vi "SCM4_MAG_Signaling.vi"() -> ()   [LabVIEW 2018]
panel:
  in  "Setpoint [T]":dbl=0.3 format="%#_4g"
  in  "Slew rate":dbl=0.3 format="%#_4g"
  in  "ico":u16(ring)=1 items=["Field"=1, "Rate"=2]
  # "ico = 1 Field\n       = 2 Rate"
  # "T/min"
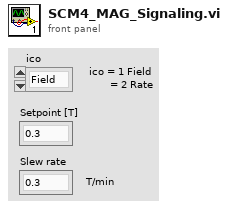
[diagram p1: front panel]
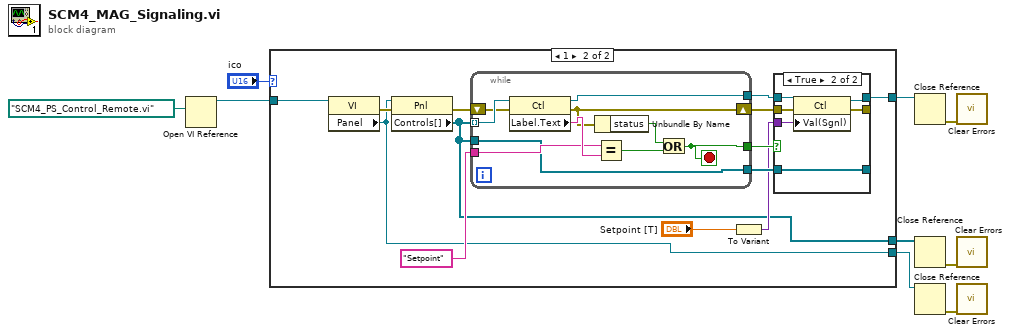
[diagram p0: block diagram]
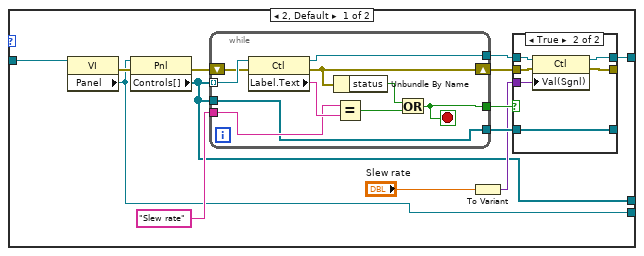
[diagram p2: hidden frame]
diagram:
  n1 = Open VI Reference(vi path=path "SCM4_PS_Control_Remote.vi") -> (vi reference=w7:refnum<vi>)  [unwired: 5 in, 1 out]
  n2 = case shown="1" "ico" {
    tunnel: w7 -> [w13 w45]
    tunnel: [w12 w44] -> w4
    tunnel: [w11 w43] -> w3
    tunnel: [w10 w42] -> w2
    frame 2, Default {
      n3 = property class="VI"(reference=w13) -> (error out=w22:errorcluster, "Panel"=w10:refnum<vi>)  [unwired: 1 in, 1 out]
      n4 = property class="Pnl"(reference=w10, error in=w22) -> (error out=w21:errorcluster, "Controls[]"=w11:refnum<vi>[])  [unwired: 1 out]
      n5 = while {
        tunnel: w11 -> [w41] mode=indexing
        tunnel: "Slew rate" ("Control Name") -> [w39]
        shift-right: [w36] -> w18
        shift-left: w21 -> [w38]
        tunnel: [w37] -> w20
        tunnel: [w33] -> w19
        tunnel: w11 -> [w32]
        tunnel: [w32] -> w17
        stop <- w33 stop-if-true
        n6 = property class="Ctl"(reference=w41, error in=w38) -> (reference out=w37:refnum<vi>, error out=w36:errorcluster, "Label.Text"=w40:string)
        n7 = Unbundle By Name(w36) -> ("status"=w35:bool)
        n8 = Equal?(x=w39, y=w40) -> (x = y?=w34:bool)
        n9 = Or(x=w35, y=w34) -> (x .or. y?=w33:bool)
      }
      n10 = To Variant(anything="Slew rate") -> (Variant=w15:variant)
      n11 = case shown="True" w19 {
        tunnel: w20 -> [w24 w30]
        tunnel: w18 -> [w25 w31]
        tunnel: [w25 w29] -> _
        tunnel: [w24 w28] -> w12
        tunnel: w17 -> [w23 w27]
        tunnel: [w23 w27] -> _
        tunnel: w15 -> [_ w26]
        frame False {
        }
        frame True {
          n12 = property on="Property Node" class="Ctl"(reference=w30, error in=w31, "Val(Sgnl)"=w26) -> (reference out=w28:refnum<vi>, error out=w29:errorcluster)
        }
      }
    }
    frame 1 {
      n13 = property class="VI"(reference=w45) -> (error out=w54:errorcluster, "Panel"=w42:refnum<vi>)  [unwired: 1 in, 1 out]
      n14 = property class="Pnl"(reference=w42, error in=w54) -> (error out=w53:errorcluster, "Controls[]"=w43:refnum<vi>[])  [unwired: 1 out]
      n15 = while {
        tunnel: w43 -> [w73] mode=indexing
        tunnel: "Setpoint" ("Control Name") -> [w71]
        shift-right: [w68] -> w50
        shift-left: w53 -> [w70]
        tunnel: [w69] -> w52
        tunnel: [w65] -> w51
        tunnel: w43 -> [w64]
        tunnel: [w64] -> w49
        stop <- w65 stop-if-true
        n16 = property class="Ctl"(reference=w73, error in=w70) -> (reference out=w69:refnum<vi>, error out=w68:errorcluster, "Label.Text"=w72:string)
        n17 = Unbundle By Name(w68) -> ("status"=w67:bool)
        n18 = Equal?(x=w71, y=w72) -> (x = y?=w66:bool)
        n19 = Or(x=w67, y=w66) -> (x .or. y?=w65:bool)
      }
      n20 = To Variant(anything="Setpoint [T]") -> (Variant=w47:variant)
      n21 = case shown="True" w51 {
        tunnel: w52 -> [w56 w62]
        tunnel: w50 -> [w57 w63]
        tunnel: [w57 w61] -> _
        tunnel: [w56 w60] -> w44
        tunnel: w49 -> [w55 w59]
        tunnel: [w55 w59] -> _
        tunnel: w47 -> [_ w58]
        frame False {
        }
        frame True {
          n22 = property class="Ctl"(reference=w62, error in=w63, "Val(Sgnl)"=w58) -> (reference out=w60:refnum<vi>, error out=w61:errorcluster)
        }
      }
    }
  }
  n23 = Close Reference(reference=w4) -> (error out=w8:errorcluster)  [unwired: 1 in]
  n24 = Close Reference(reference=w3) -> (error out=w6:errorcluster)  [unwired: 1 in]
  n25 = Close Reference(reference=w2) -> (error out=w5:errorcluster)  [unwired: 1 in]
  n26 = call <vilib>:"Clear Errors.vi"("error in (no error)"=w8) -> ()  [unwired: 5 in, 2 out]
  n27 = call <vilib>:"Clear Errors.vi"("error in (no error)"=w6) -> ()  [unwired: 5 in, 2 out]
  n28 = call <vilib>:"Clear Errors.vi"("error in (no error)"=w5) -> ()  [unwired: 5 in, 2 out]
